vi "Reset Totalizer.vi"(7 "Unit ID (A)":string="A", 8 "error in":errorcluster, 11 "VISA Session In":refnum<visa-resource-name>="Alicat") -> (0 "error out":errorcluster, 2 "Data string returned":string, 3 "VISA Session Out":refnum<visa-resource-name>)   [LabVIEW 2023]
doc: "Performs a reset of the totalizer."
uses:
  <vilib>/Instr/_visa.llb/VISA Flush IO Buffer Mask.ctl
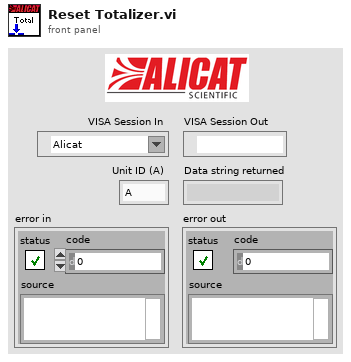
[diagram p1: front panel]
types:
  T1 = typedef "VISA Flush IO Buffer Mask.ctl" = u16
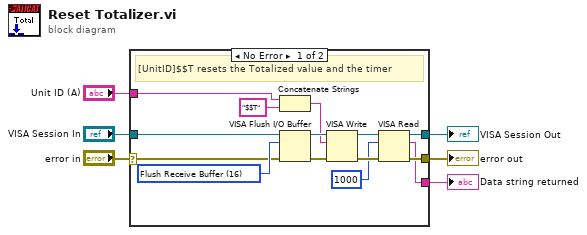
[diagram p0: block diagram]
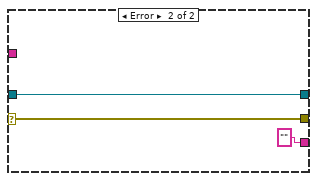
[diagram p2: hidden frame]
diagram:
  n1 = case shown="No Error" "error in" {
    selector: "error in" -> [w8 w22]
    tunnel: "VISA Session In" -> [w20 w23]
    tunnel: [w19 w23] -> w5
    tunnel: [w18 w22] -> w4
    tunnel: "Unit ID (A)" -> [w11 _]
    tunnel: [w7 "" ("read buffer")] -> w1
    frame No Error {
      w13 = T1 16 items=["Flush Receive Buffer"=16, "Write Transmit Buffer to Device"=32, "Flush Receive Buffer (No I/O)"=64, "Flush Transmit Buffer"=128] ("Mask")
      # "[UnitID]$$T resets the Totalized value and the timer"
      n2 = Concatenate Strings(w11, "$$T" ("string")) -> (w10:string)
      n3 = VISA Flush I/O Buffer(VISA resource name=w20, mask (16)=w13, error in (no error)=w8) -> (VISA resource name out=w16:refnum<visa-resource-name>, error out=w9:errorcluster)
      n4 = VISA Write(VISA resource name=w16, write buffer=w10, error in (no error)=w9) -> (VISA resource name out=w15:refnum<visa-resource-name>, error out=w17:errorcluster)  [unwired: 1 out]
      n5 = VISA Read(VISA resource name=w15, byte count=u32 1000, error in (no error)=w17) -> (VISA resource name out=w19:refnum<visa-resource-name>, read buffer=w7:string, error out=w18:errorcluster)  [unwired: 1 out]
    }
    frame Error {
    }
  }
  "error out" <- w4
  "VISA Session Out" <- w5
  "Data string returned" <- w1
